vi "SetValue.vi"(8 "error in":errorcluster, 10 "Value":bool, 11 "BooleanMeasure in":refnum<class "BooleanMeasure.lvclass">) -> (0 "error out":errorcluster, 3 "BooleanMeasure out":refnum<class "BooleanMeasure.lvclass">)   [LabVIEW 2021, in "ProligentXMLGenerator.lvlib" / "BooleanMeasure.lvclass"]
doc: "Defines the value acquired by the measure."
uses:
  BooleanMeasure.lvclass
  BooleanMeasure.lvclass/BooleanMeasure.ctl
  Base/String_4000/String_4000.lvclass
  Base/Boolean/Boolean.lvclass
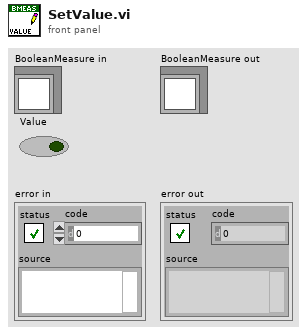
[diagram p1: front panel]
types:
  T1 = typedef "ProligentXMLGenerator.lvlib/BooleanMeasure.lvclass/Data.ctl" = cluster{"Value":refnum<class "Boolean.lvclass">}
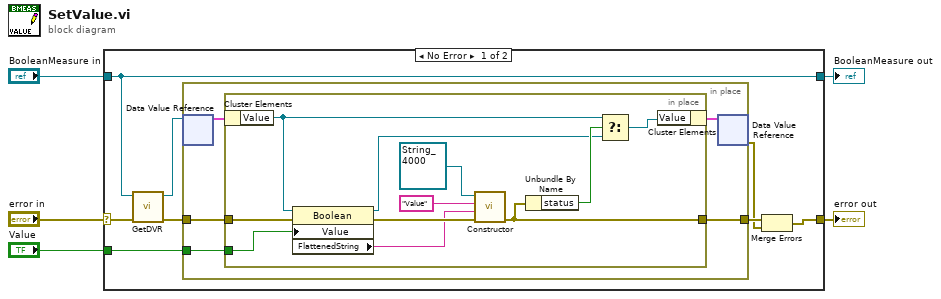
[diagram p0: block diagram]
diagram:
  n1 = case shown="No Error" "error in" {
    selector: "error in" -> [w9 w30]
    tunnel: "BooleanMeasure in" -> [w10 w31]
    tunnel: [w12 w30] -> w3
    tunnel: "Value" -> [w11 _]
    tunnel: [w10 w31] -> w1
    frame No Error {
      n2 = call "GetDVR.vi"("error in"=w9, "BooleanMeasure"=w10) -> ("error out"=w8:errorcluster, "DVRReference"=w13:refnum<data-value>)  [unwired: 8 in]
      n3 = in-place "In Place Element Structure" {
        in-place-border: w11 -> [w17]
        in-place-border: w8 -> [w18]
        in-place-border: [w16] -> w7
        n4 = in-place-dvr #1(w13) -> (w15:T1)  [unwired: 1 out]
        n5 = in-place "In Place Element Structure" {
          in-place-border: w18 -> [w29]
          in-place-border: w17 -> [w28]
          in-place-border: [w22] -> w16
          n6 = in-place-cluster #2(w15) -> ("Value"=w21:refnum<class "Boolean.lvclass">)
          n7 = property on="Property Node" class="Boolean"(reference=w21, error in=w29, "Value"=w28) -> (reference out=w20:refnum<class "Boolean.lvclass">, error out=w25:errorcluster, "FlattenedString"=w24:string)
          n8 = call-dynamic "Constructor.vi"("error in"=w25, "Value"=w24, "Name"="Value", "String in"=refnum<class "String_4000.lvclass"> refnum ("ProligentResultProcessor:String_4000")) -> ("error out"=w22:errorcluster)  [unwired: 6 in, 1 out]
          n9 = Unbundle By Name(w22) -> ("status"=w23:bool)
          n10 = Select(t=w21, s=w23, f=w20) -> (s? t:f=w19:refnum<class "Boolean.lvclass">)
          n11 = in-place-cluster #2("Value"=w19) -> (w14:T1)
        }
        n12 = in-place-dvr #1(w14) -> (w6:errorcluster)  [unwired: 1 out]
      }
      n13 = Merge Errors(w7, w6) -> (w12:errorcluster)
    }
    frame Error {
    }
  }
  "error out" <- w3
  "BooleanMeasure out" <- w1
